vi "End of Line Constant (bug fix)_csm.vi"() -> (1 "Platform EOL":string)   [LabVIEW 2020, in "Communicable State Machine.lvlib"]
uses:
  Communicable State Machine.lvlib
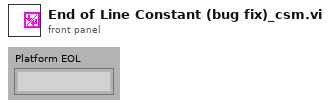
[diagram p1: front panel]
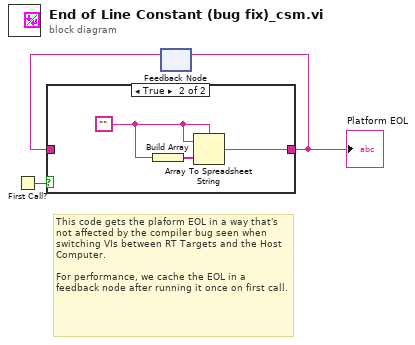
[diagram p0: block diagram]
diagram:
  # "This code gets the plaform EOL in a way that's not affected by the compiler bug seen when switching VIs between RT Targets and the Host Computer.\n\nFor performance, we cache the EOL in a feedback node after running it once on first call."
  n1 = First Call?() -> (First Call?: T/F=w1:bool)
  n2 = feedback #1() -> (w2:string)  [unwired: 1 in]
  n3 = case shown="True" w1 {
    tunnel: [w4 w5] -> w3
    tunnel: w2 -> [w4 _]
    frame False {
    }
    frame True {
      w6 = "" ("Empty String\n(hidden on FP)")
      n4 = Build Array(w6) -> (w7:string[])
      n5 = Array To Spreadsheet String(delimiter (Tab)=w6, array=w7, 3:w6) -> (spreadsheet string=w5:string)
    }
  }
  "Platform EOL" <- w3
  n6 = feedback-in #1(w3) -> ()
